vi "SetSoftwareLimits.vi"(8 "error in (no error)":errorcluster, 10 "Axis or Vector Space":u16(ring)=1 items=["Axis 1"=1, "Axis 2"=2, "Axis 3"=3, "Axis 4"=4, "Axis 5"=5, "Axis 6"=6, "Axis 7"=7, "Axis 8"=8, "Vector Space 1"=17, "Vector Space 2"=18, "Vector Space 3"=19, "Vector Space 4"=20], 11 "Board ID":u8=1 min=1 max=32 step=1) -> (0 "error out":errorcluster, 2 "Resource Output":u16(ring)=1 items=["Axis Control"=0, "Axis 1"=1, "Axis 2"=2, "Axis 3"=3, "Axis 4"=4, "Axis 5"=5, "Axis 6"=6, "Axis 7"=7, "Axis 8"=8, "Vector Space Control"=16, "Vector Space 1"=17, "Vector Space 2"=18, "Vector Space 3"=19, "Vector Space 4"=20, "Encoder Control"=32, "Encoder 1"=33, "Encoder 2"=34, "Encoder 3"=35, "Encoder 4"=36, "Encoder 5"=37, "Encoder 6"=38, "Encoder 7"=39, "Encoder 8"=40, "DAC Channel 1"=49, "DAC Channel 2"=50, "DAC Channel 3"=51, "DAC Channel 4"=52, "DAC Channel 5"=53, "DAC Channel 6"=54, "DAC Channel 7"=55, "DAC Channel 8"=56, "Stepper Output 1"=65, "Stepper Output 2"=66, "Stepper Output 3"=67, "Stepper Output 4"=68, "Stepper Output 5"=69, "Stepper Output 6"=70, "Stepper Output 7"=71, "Stepper Output 8"=72, "ADC Channel 1"=81, "ADC Channel 2"=82, "ADC Channel 3"=83, "ADC Channel 4"=84, "ADC Channel 5"=85, "ADC Channel 6"=86, "ADC Channel 7"=87, "ADC Channel 8"=88], 3 "Bd ID Out":u8)   [LabVIEW 2022 SP3]
uses:
  <vilib>/Motion/FlexMotion/FunctionsVIs/StartStopMotion.llb/Stop Motion (8 axes).flx
  <vilib>/Motion/FlexMotion/FunctionsVIs/StartStopMotion.llb/Start Motion (8 axes).flx
  <vilib>/Motion/FlexMotion/FunctionsVIs/MotionIO.llb/Enable Limits (8 axes).flx
  <vilib>/Motion/FlexMotion/CustomControls/CustomControls.llb/Axis # (8 axes).flx
  <vilib>/Motion/FlexMotion/CustomControls/CustomControls.llb/AxisOrVectorSpace To Configure.flx
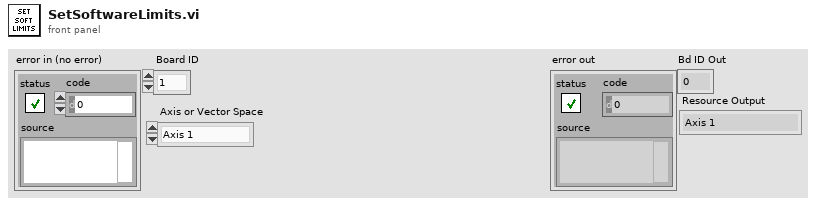
[diagram p1: front panel]
types:
  T1 = enum16{"Absolute Position", "Relative Position", "Velocity", "Relative to Cap Pos", "Modulus Position", "Absolute Contouring", "Relative Contouring"}
  T2 = typedef "Axis # (8 axes).flx" = cluster{"1":bool, "2":bool, "3":bool, "4":bool, "5":bool, "6":bool, "7":bool, "8":bool}
  T3 = typedef "AxisOrVectorSpace To Configure.flx" = u16
  T4 = typedef "Bd Id Out" = u8
  T5 = typedef "Resource Out (Enum).flx" = u16
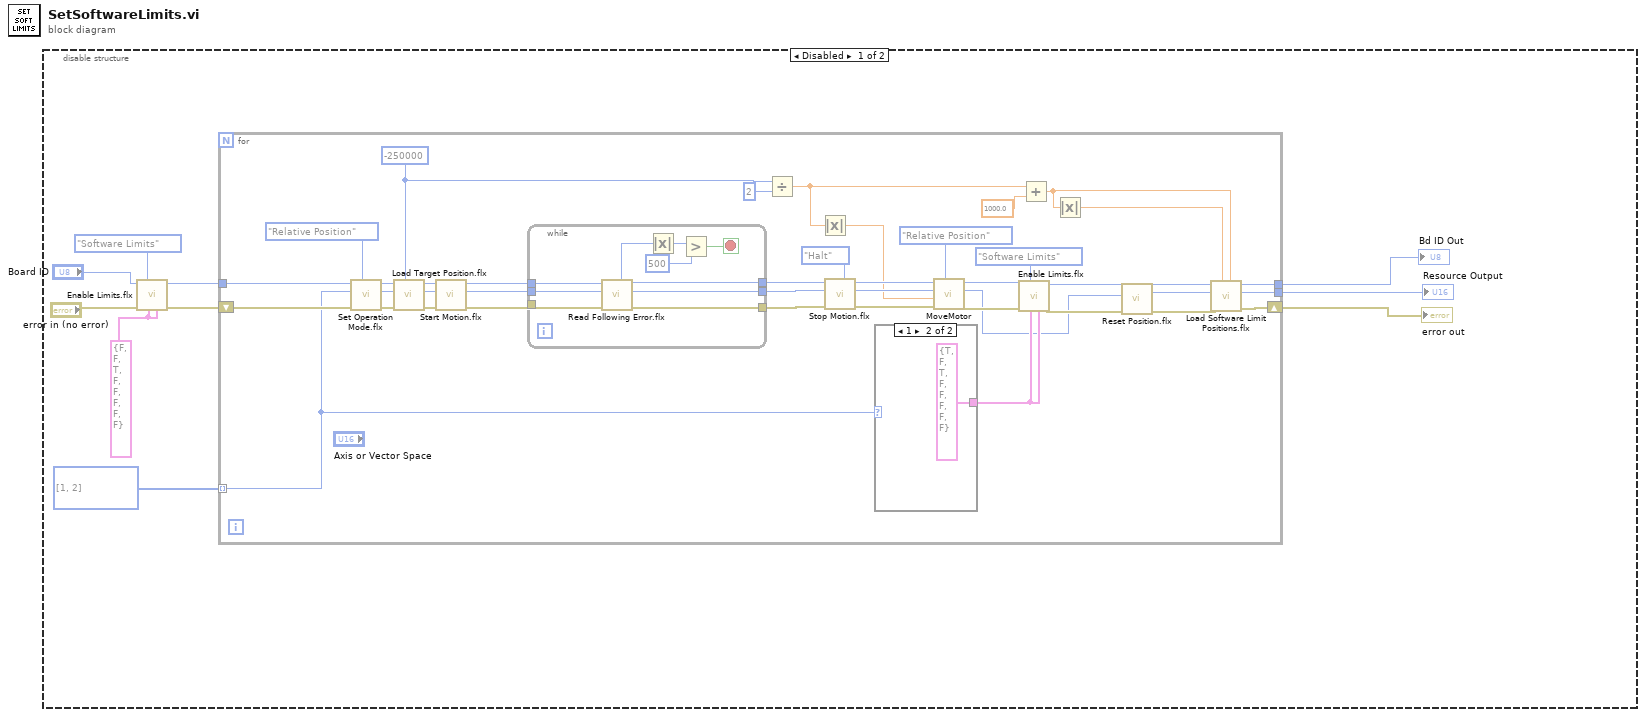
[diagram p0: block diagram]
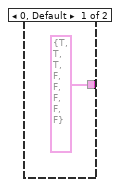
[diagram p2: hidden frame]
diagram:
  n1 = disable-structure shown="Disabled" {
    frame Disabled {
      w1 = T3[] [1, 2] items=["Axis 1"=1, "Axis 2"=2, "Axis 3"=3, "Axis 4"=4, "Axis 5"=5, "Axis 6"=6, "Axis 7"=7, "Axis 8"=8, "Vector Space 1"=17, "Vector Space 2"=18, "Vector Space 3"=19, "Vector Space 4"=20]
      w6 = T2 {"1"=FALSE, "2"=FALSE, "3"=TRUE, "4"=FALSE, "5"=FALSE, "6"=FALSE, "7"=FALSE, "8"=FALSE} ("Forward Limits (Disabled)")
      n2 = call-poly <vilib>:"Enable Limits.flx"("Reverse Limit (Disabled)"=w6, "Forward Limits (Disabled)"=w6, "Limit Type (Limit Inputs)"=enum16{"Limit Inputs", "Software Limits"}."Software Limits", "error in (no error)"="error in (no error)", "Board ID"="Board ID") -> ("error out"=w3:errorcluster, "Bd ID Out"=w2:T4)  [unwired: 5 in]
      n3 = for {
        tunnel: [w21] -> w9
        tunnel: [w20] -> w8
        tunnel: w2 -> [w18]
        shift-right: [w22] -> w10
        shift-left: w3 -> [w19]
        tunnel: w1 -> [w17] mode=indexing
        w33 = -250000 ("Target Position (0)")
        n4 = call <vilib>:"Set Operation Mode.flx"("Position Mode (Absolute)"=T1."Relative Position", "error in (no error)"=w19, "Axis or Vector Space"=w17, "Board ID"=w18) -> ("error out"=w41:errorcluster, "Resource Output"=w39:T5, "Bd ID Out"=w43:T4)  [unwired: 2 out]
        n5 = call <vilib>:"Load Target Position.flx"("Target Position (0)"=w33, "error in (no error)"=w41, "Axis"=w39, "Board ID"=w43) -> ("error out"=w40:errorcluster, "Resource Output"=w38:T5, "Bd ID Out"=w42:T4)  [unwired: 3 out]
        n6 = call-poly <vilib>:"Start Motion.flx"("error in (no error)"=w40, "Axis or Vector Space"=w38, "Board ID"=w42) -> ("error out"=w36:errorcluster, "Resource Output"=w34:T5, "Bd ID Out"=w37:T4)  [unwired: 1 in, 2 out]
        n7 = while {
          tunnel: w37 -> [w63]
          tunnel: w36 -> [w62]
          tunnel: [w57] -> w51
          tunnel: [w56] -> w50
          tunnel: [w55] -> w49
          tunnel: w34 -> [w54]
          stop <- w59 stop-if-true
          n8 = call <vilib>:"Read Following Error.flx"("error in (no error)"=w62, "Axis or Vector Space"=w54, "Board Id"=w63) -> ("error out"=w55:errorcluster, "Resource Output"=w57:T5, "Bd Id Out"=w56:T4, "Following Error"=w61:i16)  [unwired: 3 in]
          n9 = Absolute Value(x=w61) -> (abs(x)=w60:i16)
          n10 = Greater?(x=w60, y=i16 500) -> (0:w59:bool)
        }
        n11 = Divide(x=w33, y=2) -> (x/y=w30:dbl)
        n12 = Absolute Value(x=w30) -> (abs(x)=w31:dbl)
        n13 = call-poly <vilib>:"Stop Motion.flx"("Stop Type (Decel)"=enum16{"Decelerate", "Halt", "Kill"}."Halt", "error in (no error)"=w49, "Axis or Vector Space"=w51, "Board ID"=w50) -> ("error out"=w45:errorcluster, "Resource Output"=w46:T5, "Bd ID Out"=w47:T4)  [unwired: 3 in]
        n14 = case shown="1" w17 {
          tunnel: [T2 {"1"=TRUE, "2"=TRUE, "3"=TRUE, "4"=FALSE, "5"=FALSE, "6"=FALSE, "7"=FALSE, "8"=FALSE} ("Forward Limits (Disabled)") T2 {"1"=TRUE, "2"=FALSE, "3"=TRUE, "4"=FALSE, "5"=FALSE, "6"=FALSE, "7"=FALSE, "8"=FALSE} ("Forward Limits (Disabled)")] -> w23
          frame 0, Default {
          }
          frame 1 {
          }
        }
        n15 = call "MoveMotor.vi"("Position Mode (Absolute)"=T1."Relative Position", "error in (no error)"=w45, "Target Position (0)"=w31, "Axis or Vector Space"=w46, "Motion Bd ID"=w47) -> ("error out"=w25:errorcluster, "Resource Output"=w11:u16, "Bd ID Out"=w26:u8)  [unwired: 4 in]
        n16 = call-poly <vilib>:"Enable Limits.flx"("Reverse Limit (Disabled)"=w23, "Forward Limits (Disabled)"=w23, "Limit Type (Limit Inputs)"=enum16{"Limit Inputs", "Software Limits"}."Software Limits", "error in (no error)"=w25, "Board ID"=w26) -> ("error out"=w15:errorcluster, "Bd ID Out"=w16:T4)  [unwired: 5 in]
        n17 = Add(x=w30, y=1000.0) -> (x+y=w27:dbl)
        n18 = Absolute Value(x=w27) -> (abs(x)=w28:dbl)
        n19 = call <vilib>:"Reset Position.flx"("error in (no error)"=w15, "Axis"=w11, "Board ID"=w16) -> ("error out"=w14:errorcluster, "Resource Output"=w12:T5, "Bd ID Out"=w13:T4)  [unwired: 4 in]
        n20 = call <vilib>:"Load Software Limit Positions.flx"("Reverse SW Limit"=w27, "Forward SW Limit"=w28, "error in (no error)"=w14, "Axis"=w12, "Board ID"=w13) -> ("error out"=w22:errorcluster, "Resource Output"=w20:T5, "Bd ID Out"=w21:T4)  [unwired: 2 in]
      }
      "error out" <- w10
      "Bd ID Out" <- w9
      "Resource Output" <- w8
    }
    frame Enabled {
    }
  }
